vi "Basic Command Structure.vi"(2 "Execute":bool=TRUE, 7 "Action Completed?":bool) -> (13 "Done Executing":bool)   [LabVIEW 2011]
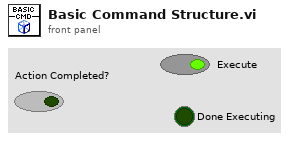
[diagram p1: front panel]
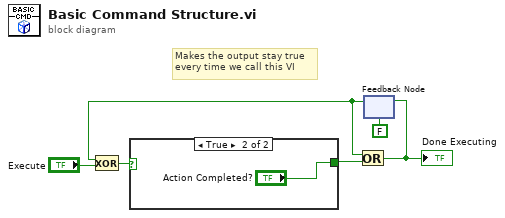
[diagram p0: block diagram]
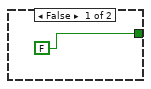
[diagram p2: hidden frame]
diagram:
  # "Makes the output stay true\nevery time we call this VI"
  n1 = feedback #1(FALSE) -> (w2:bool)
  n2 = Exclusive Or(1:"Execute", 2:w2) -> (0:w6:bool)
  n3 = case shown="True" w6 {
    tunnel: [FALSE "Action Completed?"] -> w4
    frame False {
    }
    frame True {
    }
  }
  n4 = Or(x=w2, y=w4) -> (x .or. y?=w1:bool)
  "Done Executing" <- w1
  n5 = feedback-in #1(w1) -> ()
